vi "vision acquisition 范例.vi"(5 "Stop (F)":bool, 7 "error in":errorcluster) -> (20 "Image Out":T1(plugin-control), 25 "Frame Rate":dbl, 26 "Stopped":bool, 27 "error out":errorcluster)   [LabVIEW 2017]
doc: "Creates, and edits acquisitions using the NI Vision Acquisition Express VI.\n\nThe NI Vision Acquisition Wizard is launched by placing the Express VI on the block diagram. Select an acquisition source and configure an acquisition using NI-IMAQ, NI-IMAQdx, or simulate an acquisition by reading an AVI or image files from a folder. After an acquisition is configured, select controls and indicators to be able to programmatically set in LabVIEW. Double-click the Vision Acquisition Express VI to edit the acquisition.\n\nNote: Any images created by the Express VI need to be disposed after use. Use the IMAQ Dispose.vi to cleanup the images output by the Express VI when they are no longer needed."
uses:
  <vilib>/vision/driver/NI_Vision_Acquisition_Software.lvlib
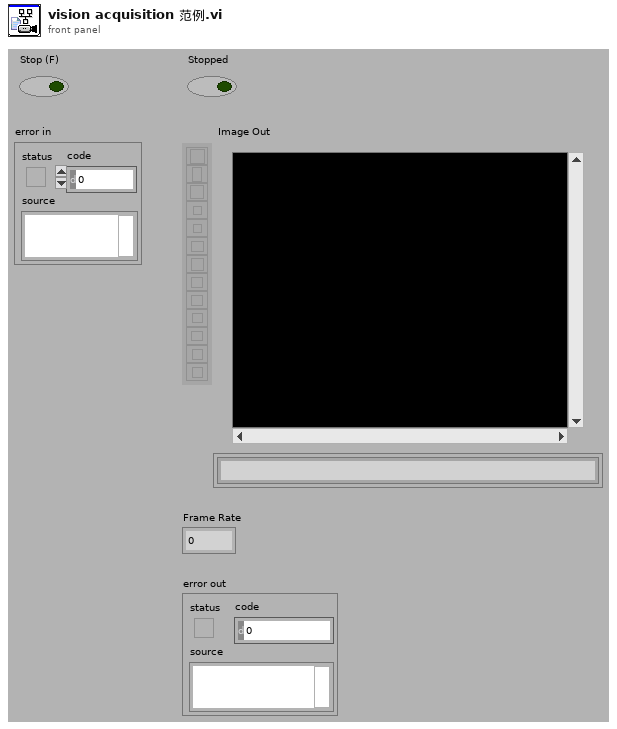
[diagram p1: front panel]
types:
  T1 = typedef "IMAQ Image.ctl" = refnum<image>
  T2 = typedef "IMAQdx.ctl" = refnum<k21>
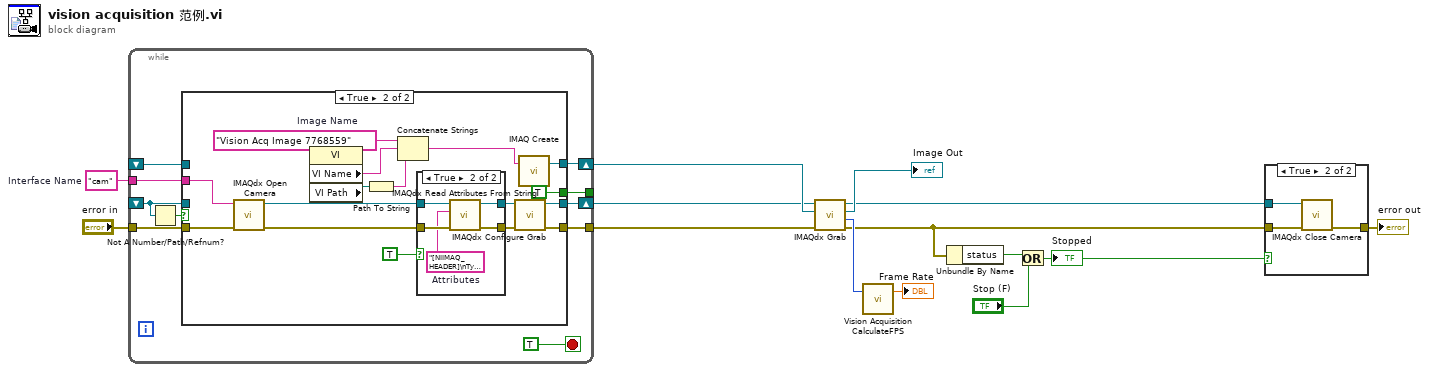
[diagram p0: block diagram]
diagram:
  w12 = "cam"  # Interface Name
  n1 = while "While Loop_template0" {
    shift-right: [w24] -> w5
    shift-left: _ -> [w17]
    tunnel: [w23] -> w13
    tunnel: "error in" -> [w22]
    shift-right: [w20] -> w6
    shift-left: _ -> [w19]
    tunnel: w12 -> [w18]
    tunnel: [w15] -> _
    stop <- TRUE ("_template0") stop-if-true
    n2 = Not A Number/Path/Refnum?(number/path/refnum=w17) -> (NaN/Path/Refnum?=w16:bool)
    n3 = case "Case Structure_template0" shown="True" w16 {
      tunnel: [w27 w42] -> w24
      tunnel: w17 -> [w27 _]
      tunnel: [w26 w41] -> w23
      tunnel: w22 -> [w26 w43]
      tunnel: [w25 w40] -> w20
      tunnel: w19 -> [w25 _]
      tunnel: w18 -> [_ w30]
      tunnel: [_ TRUE] -> w15
      frame False {
      }
      frame True {
        w35 = "Vision Acq Image 7768559"  # Image Name
        n4 = call <vilib>:"IMAQdx Open Camera.vi"("error in"=w43, "Session In"=w30) -> ("error out"=w33:errorcluster, "Session Out"=w34:T2)  [unwired: 1 in, 7 out]
        n5 = property class="VI"() -> ("VI Name"=w38:string, "VI Path"=w39:path)  [unwired: 2 in, 2 out]
        n6 = Path To String(path=w39) -> (string=w37:string)
        n7 = Concatenate Strings(w35, w38, w37) -> (w36:string)
        n8 = case "条件结构" shown="True" TRUE ("Init Attributes") {
          tunnel: w34 -> [w45 w50]
          tunnel: w33 -> [w44 w49]
          tunnel: [w45 w47] -> w32
          tunnel: [w44 w46] -> w31
          frame False {
          }
          frame True {
            w48 = "[NIIMAQ_HEADER]\nType = 2\nVersion = 8\n\n[CAMERA_DATA]\nAcquisitionAttributes::AdvancedEthernet::BandwidthControl::DesiredPeakBandwidth = \"1000\"\nAcquisitionAttributes::AdvancedEthernet::Controller::DestinationMode = \"Unicast\"\nAcquisitionAttributes::AdvancedEthernet::Controller::DestinationMulticastAddress = \"239.192.0.1\"\nAcquisitionAttributes::AdvancedEthernet::EventParameters::EventsEnabled = \"true\"\nAcquisitionAttributes::AdvancedEthernet::EventParameters::MaxOutstandingEvents = \"50\"\nAcquisitionAttributes::AdvancedEthernet::FirewallTraversal::Enabled = \"false\"\nAcquisitionAttributes::AdvancedEthernet::FirewallTraversal::KeepAliveTime = \"30\"\nAcquisitionAttributes::AdvancedEthernet::LostPacketMode = \"Ignore\"\nAcquisitionAttributes::AdvancedEthernet::ResendParameters::MaxResendsPerPacket = \"25\"\nAcquisitionAttributes::AdvancedEthernet::ResendParameters::MemoryWindowSize = \"1024\"\nAcquisitionAttributes::AdvancedEthernet::ResendParameters::MissingPacketTimeout = \"2\"\nAcquisitionAttributes::AdvancedEthernet::ResendParameters::NewPacketTimeout = \"100\"\nAcquisitionAttributes::AdvancedEthernet::ResendParameters::ResendBatchingPercentage = \"10\"\nAcquisitionAttributes::AdvancedEthernet::ResendParameters::ResendResponseTimeout = \"2\"\nAcquisitionAttributes::AdvancedEthernet::ResendParameters::ResendsEnabled = \"true\"\nAcquisitionAttributes::AdvancedEthernet::ResendParameters::ResendThresholdPercentage = \"5\"\nAcquisitionAttributes::AdvancedEthernet::ResendParameters::ResendTimerResolution = \"1\"\nAcquisitionAttributes::AdvancedEthernet::TestPacketParameters::MaxTestPacketRetries = \"1\"\nAcquisitionAttributes::AdvancedEthernet::TestPacketParameters::TestPacketEnabled = \"true\"\nAcquisitionAttributes::AdvancedEthernet::TestPacketParameters::TestPacketTimeout = \"250\"\nAcquisitionAttributes::AdvancedGenicam::CommandTimeout = \"100\"\nAcquisitionAttributes::Bayer::GainB = \"1\"\nAcquisitionAttributes::Bayer::GainG = \"1\"\nAcquisitionAttributes::Bayer::GainR = \"1\"\nAcquisitionAttributes::Bayer::Pattern = \"Use hardware value\"\nAcquisitionAttributes::BitsPerPixel = \"Use hardware value\"\nAcquisitionAttributes::ChunkDataDecoding::ChunkDataDecodingEnabled = \"false\"\nAcquisitionAttributes::ChunkDataDecoding::MaximumChunkCopySize = \"64\"\nAcquisitionAttributes::IgnoreFirstFrame = \"false\"\nAcquisitionAttributes::OverwriteMode = \"Get Newest\"\nAcquisitionAttributes::PacketSize = \"8000\"\nAcquisitionAttributes::PixelSignedness = \"Signed\"\nAcquisitionAttributes::ReceiveTimestampMode = \"None\"\nAcquisitionAttributes::ShiftPixelBits = \"false\"\nAcquisitionAttributes::SwapPixelBytes = \"false\"\nAcquisitionAttributes::Timeout = \"5000\"\nCameraAttributes::Acquisition::AcquisitionFrameCount = \"1\"\nCameraAttributes::Acquisition::AcquisitionFrameRateAbs = \"205.3388090349076\"\nCameraAttributes::Acquisition::AcquisitionMode = \"Continuous\"\nCameraAttributes::Acquisition::RecorderPreEventCount = \"0\"\nCameraAttributes::Acquisition::Trigger::TriggerSelector = \"FrameStart\"\nCameraAttributes::Acquisition::Trigger::TriggerMode = \"On\"\nCameraAttributes::Acquisition::Trigger::TriggerSource = \"Freerun\"\nCameraAttributes::Acquisition::Trigger::TriggerActivation = \"RisingEdge\"\nCameraAttributes::Acquisition::Trigger::TriggerOverlap = \"Off\"\nCameraAttributes::Acquisition::Trigger::TriggerDelayAbs = \"0\"\nCameraAttributes::Acquisition::Trigger::TriggerSelector = \"AcquisitionStart\"\nCameraAttributes::Acquisition::Trigger::TriggerMode = \"Off\"\nCameraAttributes::Acquisition::Trigger::TriggerSource = \"Line1\"\nCameraAttributes::Acquisition::Trigger::TriggerActivation = \"RisingEdge\"\nCameraAttributes::Acquisition::Trigger::TriggerSelector = \"AcquisitionEnd\"\nCameraAttributes::Acquisition::Trigger::TriggerMode = \"Off\"\nCameraAttributes::Acquisition::Trigger::TriggerSource = \"Line1\"\nCameraAttributes::Acquisition::Trigger::TriggerActivation = \"RisingEdge\"\nCameraAttributes::Acquisition::Trigger::TriggerSelector = \"AcquisitionRecord\"\nCameraAttributes::Acquisition::Trigger::TriggerMode = \"On\"\nCameraAttributes::Acquisition::Trigger::TriggerSource = \"Line1\"\nCameraAttributes::Acquisition::Trigger::TriggerActivation = \"RisingEdge\"\nCameraAttributes::Acquisition::Trigger::TriggerSelector = \"FrameStart\"\nCameraAttributes::Controls::DSPSubregion::DSPSubregionBottom = \"4294967295\"\nCameraAttributes::Controls::DSPSubregion::DSPSubregionLeft = \"0\"\nCameraAttributes::Controls::DSPSubregion::DSPSubregionRight = \"4294967295\"\nCameraAttributes::Controls::DSPSubregion::DSPSubregionTop = \"0\"\nCameraAttributes::Controls::Exposure::ExposureAuto = \"Off\"\nCameraAttributes::Controls::Exposure::ExposureAutoControl::ExposureAutoAdjustTol = \"5\"\nCameraAttributes::Controls::Exposure::ExposureAutoControl::ExposureAutoAlg = \"Mean\"\nCameraAttributes::Controls::Exposure::ExposureAutoControl::ExposureAutoMax = \"500000\"\nCameraAttributes::Controls::Exposure::ExposureAutoControl::ExposureAutoMin = \"25\"\nCameraAttributes::Controls::Exposure::ExposureAutoControl::ExposureAutoOutliers = \"0\"\nCameraAttributes::Controls::Exposure::ExposureAutoControl::ExposureAutoRate = \"100\"\nCameraAttributes::Controls::Exposure::ExposureAutoControl::ExposureAutoTarget = \"50\"\nCameraAttributes::Controls::Exposure::ExposureMode = \"Timed\"\nCameraAttributes::Controls::Exposure::ExposureTimeAbs = \"15000\"\nCameraAttributes::Controls::Gain::GainAutoControl::GainAutoAdjustTol = \"5\"\nCameraAttributes::Controls::Gain::GainAutoControl::GainAutoMax = \"24\"\nCameraAttributes::Controls::Gain::GainAutoControl::GainAutoMin = \"0\"\nCameraAttributes::Controls::Gain::GainAutoControl::GainAutoOutliers = \"0\"\nCameraAttributes::Controls::Gain::GainAutoControl::GainAutoRate = \"100\"\nCameraAttributes::Controls::Gain::GainAutoControl::GainAutoTarget = \"50\"\nCameraAttributes::Controls::Gain::GainSelector = \"All\"\nCameraAttributes::Controls::Gain::GainRaw = \"0\"\nCameraAttributes::Controls::Gain::GainAuto = \"Off\"\nCameraAttributes::EventControl::EventSelector = \"AcquisitionStart\"\nCameraAttributes::EventControl::EventNotification = \"Off\"\nCameraAttributes::EventControl::EventSelector = \"AcquisitionEnd\"\nCameraAttributes::EventControl::EventNotification = \"Off\"\nCameraAttributes::EventControl::EventSelector = \"FrameTrigger\"\nCameraAttributes::EventControl::EventNotification = \"Off\"\nCameraAttributes::EventControl::EventSelector = \"ExposureEnd\"\nCameraAttributes::EventControl::EventNotification = \"Off\"\nCameraAttributes::EventControl::EventSelector = \"AcquisitionRecordTrigger\"\nCameraAttributes::EventControl::EventNotification = \"Off\"\nCameraAttributes::EventControl::EventSelector = \"Line1RisingEdge\"\nCameraAttributes::EventControl::EventNotification = \"Off\"\nCameraAttributes::EventControl::EventSelector = \"Line1FallingEdge\"\nCameraAttributes::EventControl::EventNotification = \"Off\"\nCameraAttributes::EventControl::EventSelector = \"Line2RisingEdge\"\nCameraAttributes::EventControl::EventNotification = \"Off\"\nCameraAttributes::EventControl::EventSelector = \"Line2FallingEdge\"\nCameraAttributes::EventControl::EventNotification = \"Off\"\nCameraAttributes::EventControl::EventSelector = \"Line3RisingEdge\"\nCameraAttributes::EventControl::EventNotification = \"Off\"\nCameraAttributes::EventControl::EventSelector = \"Line3FallingEdge\"\nCameraAttributes::EventControl::EventNotification = \"Off\"\nCameraAttributes::EventControl::EventSelector = \"Line4RisingEdge\"\nCameraAttributes::EventControl::EventNotification = \"Off\"\nCameraAttributes::EventControl::EventSelector = \"Line4FallingEdge\"\nCameraAttributes::EventControl::EventNotification = \"Off\"\nCameraAttributes::EventControl::EventSelector = \"AcquisitionStart\"\nCameraAttributes::EventControl::EventsEnable1 = \"0\"\nCameraAttributes::GigE::BandwidthControlMode = \"StreamBytesPerSecond\"\nCameraAttributes::GigE::ChunkModeActive = \"false\"\nCameraAttributes::GigE::StreamBytesPerSecond = \"115000000\"\nCameraAttributes::GigE::StreamFrameRateConstrain = \"true\"\nCameraAttributes::GigE::StreamHold::StreamHoldEnable = \"Off\"\nCameraAttributes::ImageFormat::Height = \"480\"\nCameraAttributes::ImageFormat::OffsetX = \"0\"\nCameraAttributes::ImageFormat::OffsetY = \"0\"\nCameraAttributes::ImageFormat::PixelFormat = \"Mono8\"\nCameraAttributes::ImageFormat::Width = \"640\"\nCameraAttributes::ImageMode::BinningHorizontal = \"1\"\nCameraAttributes::ImageMode::BinningVertical = \"1\"\nCameraAttributes::IO::Strobe::StrobeDelay = \"0\"\nCameraAttributes::IO::Strobe::StrobeDuration = \"0\"\nCameraAttributes::IO::Strobe::StrobeDurationMode = \"Source\"\nCameraAttributes::IO::Strobe::StrobeSource = \"FrameTrigger\"\nCameraAttributes::IO::SyncIn::SyncInSelector = \"SyncIn1\"\nCameraAttributes::IO::SyncIn::SyncInGlitchFilter = \"0\"\nCameraAttributes::IO::SyncOut::SyncOutLevels = \"0\"\nCameraAttributes::IO::SyncOut::SyncOutSelector = \"SyncOut1\"\nCameraAttributes::IO::SyncOut::SyncOutSource = \"FrameTrigger\"\nCameraAttributes::IO::SyncOut::SyncOutPolarity = \"Normal\"\nCameraAttributes::IO::SyncOut::SyncOutSelector = \"SyncOut2\"\nCameraAttributes::IO::SyncOut::SyncOutSource = \"Exposing\"\nCameraAttributes::IO::SyncOut::SyncOutPolarity = \"Normal\"\nCameraAttributes::IO::SyncOut::SyncOutSelector = \"SyncOut3\"\nCameraAttributes::IO::SyncOut::SyncOutSource = \"Exposing\"\nCameraAttributes::IO::SyncOut::SyncOutPolarity = \"Normal\"\nCameraAttributes::IO::SyncOut::SyncOutSelector = \"SyncOut1\"\n"  # Attributes
            n9 = call <vilib>:"IMAQdx Read Attributes From String.vi"("error in"=w49, "Attributes String In"=w48, "Session In"=w50) -> ("error out"=w46:errorcluster, "Session Out"=w47:T2)  [unwired: 7 out]
          }
        }
        n10 = call <vilib>:"IMAQdx Configure Grab.vi"("error in"=w31, "Session In"=w32) -> ("error out"=w41:errorcluster, "Session Out"=w42:T2)  [unwired: 8 out]
        n11 = call "IMAQ Create"("Image Name"=w36) -> ("New Image"=w40:T1)  [unwired: 3 in, 2 out]
      }
    }
  }
  n12 = call <vilib>:"IMAQdx Grab.vi"("error in"=w13, "Image In"=w6, "Session In"=w5) -> ("error out"=w4:errorcluster, "Buffer Number Out"=w8:u32, "Image Out"=→"Image Out":T1, "Session Out"=w3:T2)  [unwired: 1 in, 4 out]
  n13 = call <vilib>:"Vision Acquisition CalculateFPS.vi"("buffer number"=w8) -> ("acquired FPS"=→"Frame Rate":dbl)  [unwired: 2 out]
  n14 = Unbundle By Name(w4) -> ("status"=w11:bool)
  n15 = Or(x=w11, y="Stop (F)") -> (x .or. y?=w2:bool)
  "Stopped" <- w2
  n16 = case "Case Structure_template1" shown="True" w2 {
    tunnel: [w51 w53] -> w1
    tunnel: w4 -> [w51 w54]
    tunnel: w3 -> [_ w52]
    frame False {
    }
    frame True {
      n17 = call <vilib>:"IMAQdx Close Camera.vi"("error in"=w54, "Session In"=w52) -> ("error out"=w53:errorcluster)  [unwired: 9 out]
    }
  }
  "error out" <- w1
